vi "BallSystemSelector.vi"() -> ()   [LabVIEW 2019]
uses:
  Controls/Ball System Actions.ctl
panel:
  in  "Ball System Actions":T1
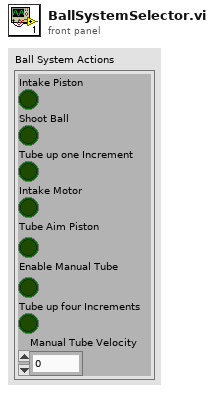
[diagram p1: front panel]
types:
  T1 = typedef "Ball System Actions.ctl" = cluster{"Intake Piston ":bool, "Shoot Ball":bool, "Tube up one Increment\t":bool, "Intake Motor\t":bool, "Tube Aim Piston":bool, "Enable Manual Tube":bool, "Tube up four Increments":bool, "Manual Tube Velocity":dbl}
  T2 = typedef "WPI_MotorControlDeviceRef.ctl" = cluster{"DeviceStatus":errorcluster, "Type":T3, "PWM":cluster{"PWM Channel":T4, "DeadBand":T5}, "CAN":cluster{"Device Number":u8, "SetOutput VI Ref":variant, "GetOutput VI Ref":variant, "Enable VI Ref":variant, "Disable VI Ref":variant, "Data":variant}, "Invert":bool, "DIO PWM":cluster{"PWM \"Enable\" Channel":T4, "DIOChannel":T6, "PWM Rate":dbl}}
  T3 = typedef "WPI_MotorControlType.ctl" = enum16{"PWM", "CAN", "DIO PWM"}
  T4 = typedef "FPGA_DIOPWMChannel.ctl" = enum8{"PWM 0", "PWM 1", "PWM 2", "PWM 3", "PWM 4", "PWM 5", "PWM 6", "PWM 7", "PWM 8", "PWM 9", "PWM MXP 0", "PWM MXP 1", "PWM MXP 2", "PWM MXP 3", "PWM MXP 4", "PWM MXP 5", "PWM MXP 6", "PWM MXP 7", "PWM MXP 8", "PWM MXP 9", "Invalid"}
  T5 = typedef "WPI_PWMDeadband.ctl" = cluster{"Name":string, "maxPositivePwm":i32, "minPositivePwm":i32, "centerPwm":i32, "maxNegativePwm":i32, "minNegativePwm":i32, "angularRange":u16}
  T6 = typedef "FPGA_DIOChannel.ctl" = enum8{"DIO 0", "DIO 1", "DIO 2", "DIO 3", "DIO 4", "DIO 5", "DIO 6", "DIO 7", "DIO 8", "DIO 9", "DIO MXP 0", "DIO MXP 1", "DIO MXP 2", "DIO MXP 3", "DIO MXP 4", "DIO MXP 5", "DIO MXP 6", "DIO MXP 7", "DIO MXP 8", "DIO MXP 9", "DIO MXP 10", "DIO MXP 11", "DIO MXP 12", "DIO MXP 13", "DIO MXP 14", "DIO MXP 15", "SPI Port CS1", "SPI Port CS2", "SPI Port CS3", "SPI Port MISO", "SPI Port MOSI", "Invalid"}
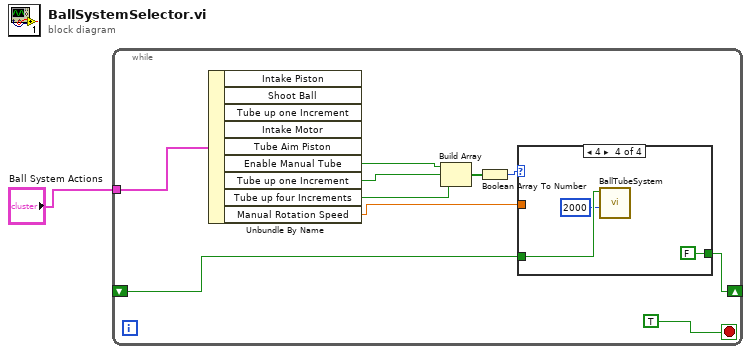
[diagram p0: block diagram]
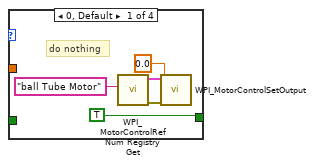
[diagram p2: hidden frame]
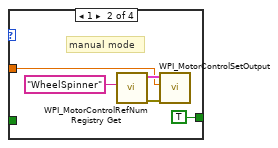
[diagram p3: hidden frame]
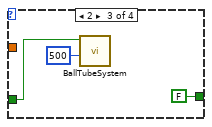
[diagram p4: hidden frame]
diagram:
  n1 = while {
    shift-right: [w8] -> _
    shift-left: _ -> [w7]
    tunnel: "Ball System Actions" -> [w2]
    stop <- TRUE stop-if-true
    n2 = Unbundle By Name(w2) -> ("Enable Manual Tube"=w6:bool, "Tube up one Increment"=w5:bool, "Tube up four Increments"=w4:bool, "Manual Rotation Speed"=w3:dbl)  [unwired: 5 out]
    n3 = Build Array(w6, w5, w4) -> (w10:bool[])
    n4 = Boolean Array To Number(Boolean array=w10) -> (number=w11:u32)
    n5 = case shown="4" w11 {
      tunnel: w3 -> [_ w18 _ _]
      tunnel: [TRUE TRUE FALSE FALSE] -> w8
      tunnel: w7 -> [_ _ w23 w26]
      frame 0, Default {
        # "do nothing"
        n6 = call <vilib>:"WPI_MotorControlRefNum Registry Get.vi"("refnum name"="ball Tube Motor") -> ("error out"=w16:errorcluster, "MotorControlDevRef"=w15:T2)  [unwired: 9 in]
        n7 = call <vilib>:"WPI_MotorControlSetOutput.vi"("error in (no error)"=w16, "Output"=0.0, "MotorControlDevRef"=w15) -> ()  [unwired: 6 in, 3 out]
      }
      frame 1 {
        # "manual mode"
        n8 = call <vilib>:"WPI_MotorControlRefNum Registry Get.vi"("refnum name"="WheelSpinner") -> ("error out"=w21:errorcluster, "MotorControlDevRef"=w20:T2)  [unwired: 9 in]
        n9 = call <vilib>:"WPI_MotorControlSetOutput.vi"("error in (no error)"=w21, "Output"=w18, "MotorControlDevRef"=w20) -> ()  [unwired: 6 in, 3 out]
      }
      frame 2 {
        n10 = call "BallTubeSystem.vi"("Duration in ms"=500, "Initialize"=w23) -> ()  [unwired: 8 in, 1 out]
      }
      frame 4 {
        n11 = call "BallTubeSystem.vi"("Duration in ms"=2000, "Initialize"=w26) -> ()  [unwired: 8 in, 1 out]
      }
    }
  }
